vi "Test_Send_Message.vi"() -> ()   [LabVIEW 2024]
doc: "This example performs writes and reads on a serial port, as directed by the user. You can press the Write and Read buttons, and change the Read Count, while the example is running.\n\nThe parameters set for the serial port must match the parameters of the connected instrument or device. In this example, the Read Count parameter specifies the number of bytes that the serial port reads. If there were more bytes at the port than the specified number, those bytes would not be read. If there were less bytes at the port than the specified number, you would receive a timeout error.\n\nThis example expands upon the flow control options for XON and XOFF, allowing the user to choose those control characters. Also, the user can enable or disable a termination character. Some devices require a termination character in order to identify the end of command strings. Some devices send a termination character to signify the end of data to be read. This example shows how you can end the Read operation once a termination character is detected in the buffer and/or append a termination character at the end of the Write data."
uses:
  <vilib>/Instr/_visa.llb/VISA Configure Serial Port (Instr).vi
panel:
  out "offset past match":i32
  out "read buffer":string
  out "Waveform Chart":dbl[][](graph)
  in  "Command List":string="stop\nencode 0\nslist 0 0\nslist 1 1\nsrate 6000\nps 2\ndec 1\ndeca 3\nnop\n"
  in  "Stop":bool
  in  "2108 CDC Virtual COM":refnum<visa-resource-name>="COM3"
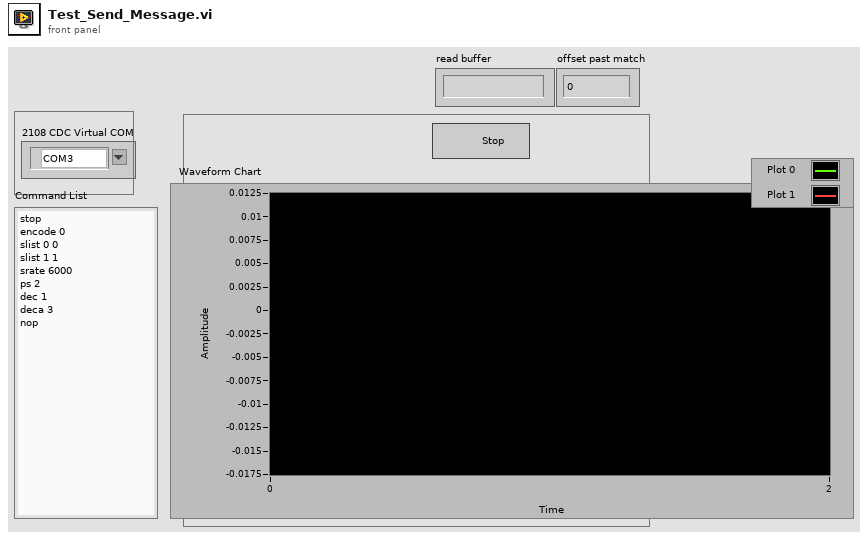
[diagram p1: front panel]
types:
  T1 = enum16{"big-endian, network order", "native, host order", "little-endian"}
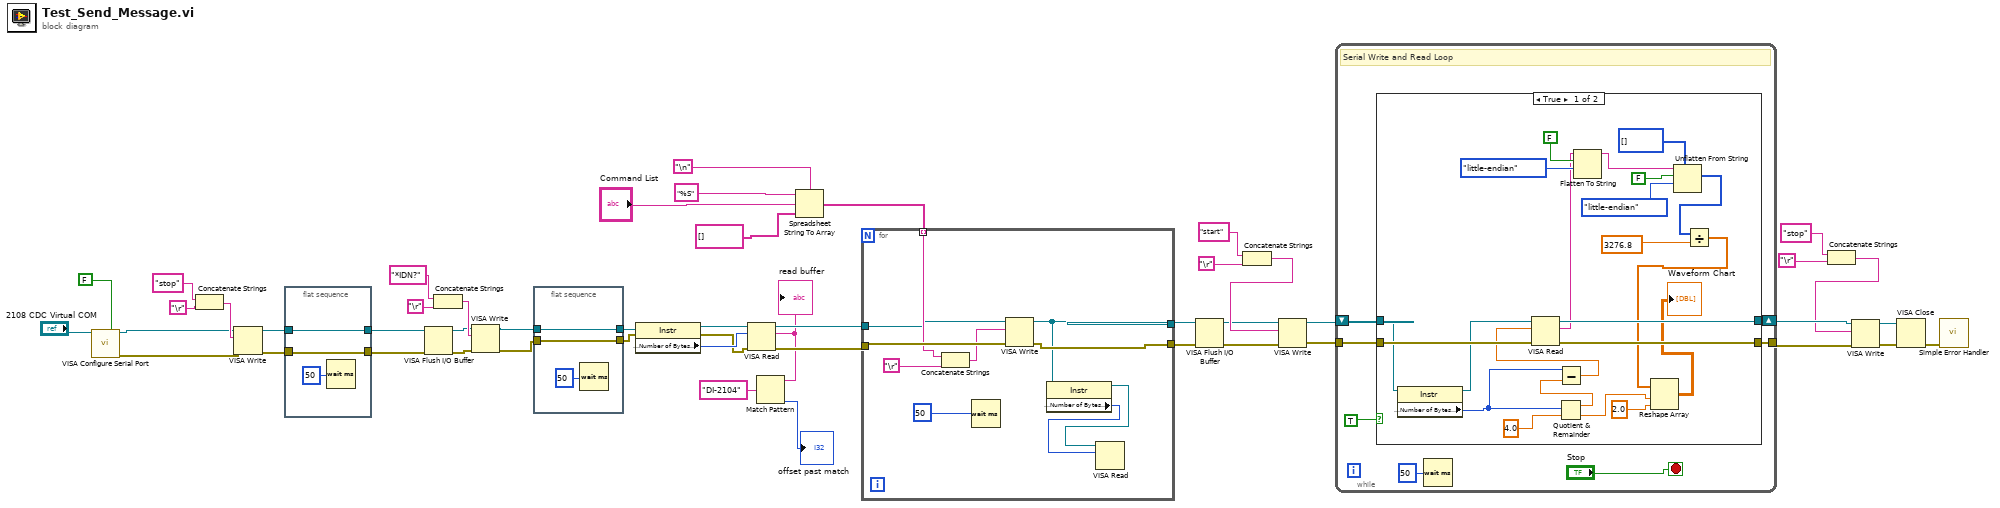
[diagram p0: block diagram]
diagram:
  n1 = call-poly "VISA Configure Serial Port"("VISA resource name"="2108 CDC Virtual COM", "Enable Termination\nChar (T)"=FALSE) -> ("VISA resource name out"=w6:refnum<visa-resource-name>, "error out"=w5:errorcluster)  [unwired: 8 in, 4 out]
  n2 = Concatenate Strings("stop", "\r") -> (w7:string)
  n3 = VISA Write(VISA resource name=w6, write buffer=w7, error in (no error)=w5) -> (VISA resource name out=w3:refnum<visa-resource-name>, error out=w2:errorcluster)  [unwired: 1 out]
  n4 = flat-sequence {
    tunnel: [w53] -> w4
    tunnel: w3 -> [w53]
    tunnel: w2 -> [w52]
    tunnel: [w52] -> w1
    frame #0 {
      n5 = Wait (ms)(milliseconds to wait=u32 50) -> ()  [unwired: 1 out]
    }
  }
  n6 = VISA Flush I/O Buffer(VISA resource name=w4, error in (no error)=w1) -> (VISA resource name out=w23:refnum<visa-resource-name>, error out=w22:errorcluster)  [unwired: 1 in]
  n7 = Concatenate Strings("*IDN?", "\r") -> (w24:string)
  n8 = VISA Write(VISA resource name=w23, write buffer=w24, error in (no error)=w22) -> (VISA resource name out=w15:refnum<visa-resource-name>, error out=w14:errorcluster)  [unwired: 1 out]
  n9 = flat-sequence {
    tunnel: [w56] -> w16
    tunnel: w15 -> [w56]
    tunnel: w14 -> [w55]
    tunnel: [w55] -> w13
    frame #0 {
      n10 = Wait (ms)(milliseconds to wait=u32 50) -> ()  [unwired: 1 out]
    }
  }
  n11 = property class="Instr"(reference=w16, error in=w13) -> (reference out=w20:refnum<visa-resource-name>, error out=w19:errorcluster, "Serial Settings:Number of Bytes at Serial Port"=w21:u32)
  n12 = VISA Read(VISA resource name=w20, byte count=w21, error in (no error)=w19) -> (VISA resource name out=w18:refnum<visa-resource-name>, read buffer=w11:string, error out=w17:errorcluster)  [unwired: 1 out]
  "read buffer" <- w11
  n13 = Match Pattern(string=w11, regular expression="DI-2104") -> (offset past match=→"offset past match":i32)  [unwired: 1 in, 3 out]
  n14 = Spreadsheet String To Array(delimiter (Tab)="\n", format string="%S", spreadsheet string="Command List", array type (2D Dbl)=string[] []) -> (array=w46:string[])
  n15 = for {
    tunnel: w46 -> [w64] mode=indexing
    tunnel: w17 -> [w66]
    tunnel: [w60] -> w30
    tunnel: [w61] -> w28
    tunnel: w18 -> [w57]
    n16 = Concatenate Strings(w64, "\r") -> (w62:string)
    n17 = Wait (ms)(milliseconds to wait=u32 50) -> ()  [unwired: 1 out]
    n18 = VISA Write(VISA resource name=w57, write buffer=w62, error in (no error)=w66) -> (VISA resource name out=w60:refnum<visa-resource-name>, error out=w61:errorcluster)  [unwired: 1 out]
    n19 = property class="Instr"(reference=w60) -> (reference out=w59:refnum<visa-resource-name>, "Serial Settings:Number of Bytes at Serial Port"=w58:u32)  [unwired: 1 in, 1 out]
    n20 = VISA Read(VISA resource name=w59, byte count=w58) -> ()  [unwired: 1 in, 4 out]
  }
  n21 = VISA Flush I/O Buffer(VISA resource name=w30, error in (no error)=w28) -> (VISA resource name out=w29:refnum<visa-resource-name>, error out=w27:errorcluster)  [unwired: 1 in]
  n22 = Concatenate Strings("start", "\r") -> (w34:string)
  n23 = VISA Write(VISA resource name=w29, write buffer=w34, error in (no error)=w27) -> (VISA resource name out=w33:refnum<visa-resource-name>, error out=w32:errorcluster)  [unwired: 1 out]
  n24 = while {
    shift-right: [w73] -> w43
    shift-left: w33 -> [w69]
    tunnel: w32 -> [w68]
    tunnel: [w71] -> w40
    stop <- "Stop" stop-if-true
    # "Serial Write and Read Loop"
    n25 = case shown="True" TRUE {
      tunnel: [w94 w97] -> w73
      tunnel: w69 -> [w92 w97]
      tunnel: w68 -> [w95 w96]
      tunnel: [w87 w96] -> w71
      frame True {
        n26 = property class="Instr"(reference=w92) -> (reference out=w86:refnum<visa-resource-name>, "Serial Settings:Number of Bytes at Serial Port"=w91:u32)  [unwired: 1 in, 1 out]
        n27 = Quotient & Remainder(x=w91, y=4.0) -> (x-y*floor(x/y)=w89:dbl, floor(x/y)=w75:dbl)
        n28 = Subtract(x=w91, y=w89) -> (x-y=w88:dbl)
        n29 = VISA Read(VISA resource name=w86, byte count=w88, error in (no error)=w95) -> (VISA resource name out=w94:refnum<visa-resource-name>, read buffer=w80:string, error out=w87:errorcluster)  [unwired: 1 out]
        n30 = Flatten To String(anything=w80, prepend array or string size? (T)=FALSE, byte order (0:big-endian, network order)=T1."little-endian") -> (data string=w81:string)  [unwired: 1 in, 2 out]
        n31 = Unflatten From String(type=i16[] [], binary string=w81, data includes array or string size? (T)=FALSE, byte order (0:big-endian, network order)=T1."little-endian") -> (value=w79:i16[])  [unwired: 1 in, 2 out]
        n32 = Divide(x=w79, y=3276.8) -> (x/y=w77:dbl[])
        n33 = Reshape Array(w77, w75, 2.0) -> (→"Waveform Chart":dbl[][])
      }
      frame False {
      }
    }
    n34 = Wait (ms)(milliseconds to wait=u32 50) -> ()  [unwired: 1 out]
  }
  n35 = Concatenate Strings("stop", "\r") -> (w37:string)
  n36 = VISA Write(VISA resource name=w43, write buffer=w37, error in (no error)=w40) -> (VISA resource name out=w42:refnum<visa-resource-name>, error out=w41:errorcluster)  [unwired: 1 out]
  n37 = VISA Close(VISA resource name=w42, error in (no error)=w41) -> (error out=w50:errorcluster)
  n38 = call <vilib>:"Simple Error Handler.vi"("error in (no error)"=w50) -> ()  [unwired: 1 in, 8 out]
